vi "Write Focus by Mode.vi"(8 "error in (no error)":errorcluster, 10 "Focus by Mode":T1, 11 "Instrument in":refnum<class "Instrument.lvclass">) -> (0 "error out":errorcluster, 3 "Instrument out":refnum<class "Instrument.lvclass">)   [LabVIEW 2018, in "Instrument.lvclass"]
uses:
  Instrument.lvclass
  Instrument.lvclass/Instrument.ctl
panel:
  out "Focus by Mode.Instrumental \npolarization":dbl
  out "Focus by Mode.Polarimetry \nEfficiency":dbl
  out "Focus by Mode.Polarimetry":dbl
  out "Focus by Mode.Photometric":dbl
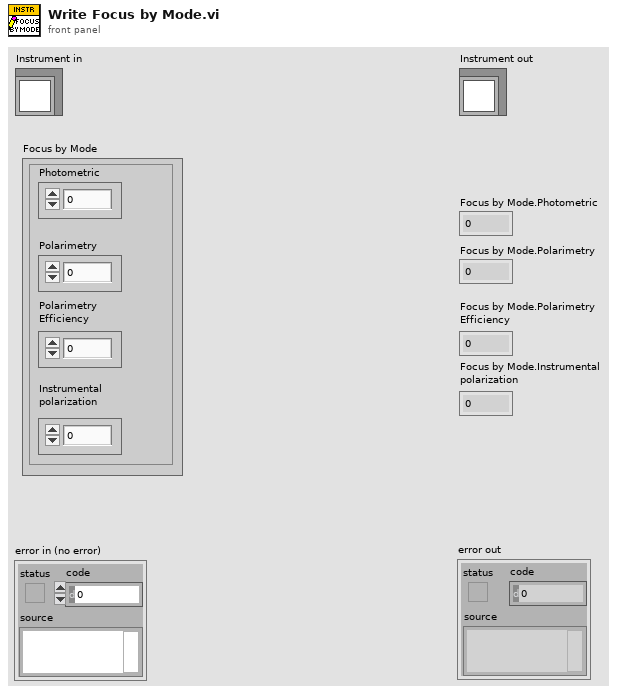
[diagram p1: front panel]
types:
  T1 = cluster{"Photometric":dbl, "Polarimetry":dbl, "Polarimetry \nEfficiency":dbl, "Instrumental  \npolarization":dbl}
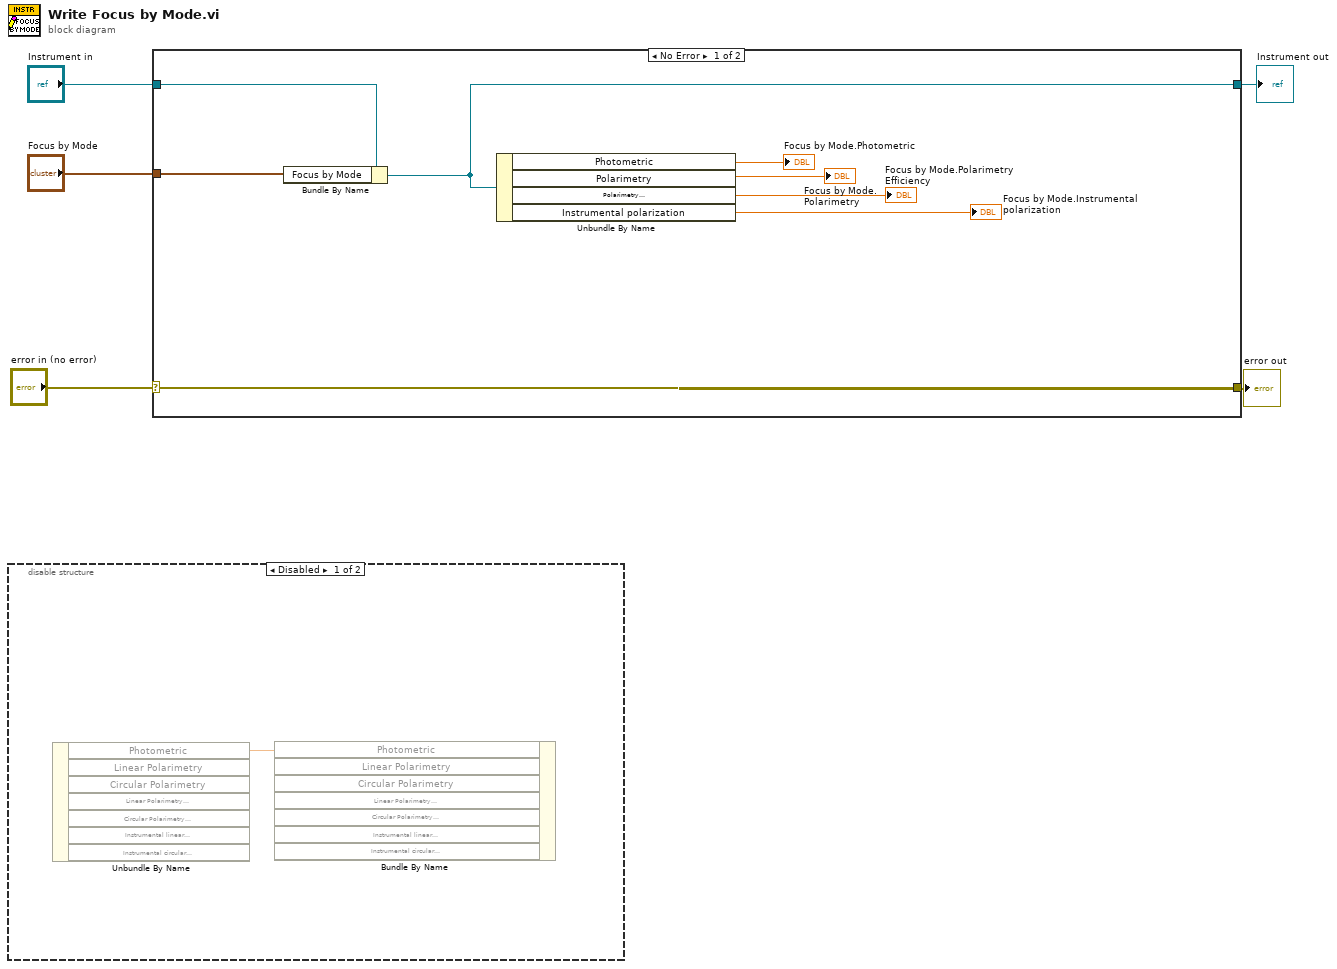
[diagram p0: block diagram]
diagram:
  n1 = disable-structure shown="Disabled" {
    frame Disabled {
      n2 = Unbundle By Name() -> ("Photometric"=w6:dbl)  [unwired: 1 in, 6 out]
      n3 = Bundle By Name("Photometric"=w6) -> (w7:cluster{})  [unwired: 6 in, 1 out]
    }
    frame Enabled {
    }
  }
  n4 = case shown="No Error" "error in (no error)" {
    selector: "error in (no error)" -> [w15 w16]
    tunnel: [w15 w16] -> w4
    tunnel: [w11 w17] -> w2
    tunnel: "Instrument in" -> [w14 w17]
    tunnel: "Focus by Mode" -> [w12 _]
    frame No Error {
      n5 = Bundle By Name(cluster=w14, "Focus by Mode"=w12) -> (w11:refnum<class "Instrument.lvclass">)
      n6 = Unbundle By Name(w11) -> ("Photometric"=→"Focus by Mode.Photometric":dbl, "Polarimetry"=→"Focus by Mode.Polarimetry":dbl, "Polarimetry \nEfficiency"=→"Focus by Mode.Polarimetry \nEfficiency":dbl, "Instrumental polarization"=→"Focus by Mode.Instrumental \npolarization":dbl)
    }
    frame Error {
    }
  }
  "error out" <- w4
  "Instrument out" <- w2
